vi "_write_yokogawa.vi"(2 "error in":errorcluster, 3 "write buffer":string) -> (0 "error out":errorcluster)   [LabVIEW 2013]
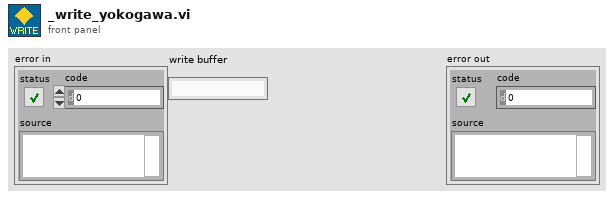
[diagram p1: front panel]
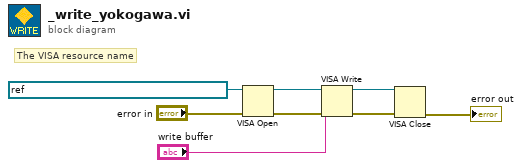
[diagram p0: block diagram]
diagram:
  # "The VISA resource name"
  n1 = VISA Open(error in (no error)="error in", VISA resource name=refnum<visa-resource-name> "USB::0xB21::0x39::91NA15589::INSTR") -> (VISA resource name=w7:refnum<visa-resource-name>, error out=w6:errorcluster)  [unwired: 3 in]
  n2 = VISA Write(VISA resource name=w7, write buffer="write buffer", error in (no error)=w6) -> (VISA resource name out=w4:refnum<visa-resource-name>, error out=w3:errorcluster)  [unwired: 1 out]
  n3 = VISA Close(VISA resource name=w4, error in (no error)=w3) -> (error out=→"error out":errorcluster)
